vi "Autonomous Independent.vi"   [LabVIEW 2016]
doc: "This VI is called when autonomous begins, and will automatically be terminated when autonomous ends. You can carry out timed or sensor driven robot movement independently without needing to return to the caller."
uses:
  <vilib>/Rock Robotics/WPI/Utilities/WPI_GetSetVariantRefNum.vi
  <vilib>/Rock Robotics/Network Tables/NT Read String.vi
  <vilib>/Rock Robotics/Network Tables/NT Write Numeric Array.vi
panel:
  # "Be sure to right-click and choose Data Operations>>Make Current Value default if you want to save the array values with the VI"
types:
  T1 = typedef "WPI_JoystickDevRef.ctl" = cluster{"Device":T2}
  T2 = typedef "WPI_JoystickDeviceEnum.ctl" = enum16{"USB 0", "USB 1", "USB 2", "USB 3", "USB 4", "USB 5"}
  T3 = typedef "WPI_RobotDriveDevRef.ctl" = cluster{"DevStatus":errorcluster, "Motors[]":T4[], "Square Inputs":bool, "Max Output":dbl}
  T4 = typedef "WPI_MotorControlDeviceRef.ctl" = cluster{"DeviceStatus":errorcluster, "Type":T5, "PWM":cluster{"PWM Channel":T6, "DeadBand":T7}, "CAN":cluster{"Device Number":u8, "SetOutput VI Ref":variant, "GetOutput VI Ref":variant, "Enable VI Ref":variant, "Disable VI Ref":variant, "Data":variant}, "Invert":bool}
  T5 = typedef "WPI_MotorControlType.ctl" = enum16{"PWM", "CAN"}
  T6 = typedef "FPGA_DIOPWMChannel.ctl" = enum8{"PWM 0", "PWM 1", "PWM 2", "PWM 3", "PWM 4", "PWM 5", "PWM 6", "PWM 7", "PWM 8", "PWM 9", "PWM MXP 0", "PWM MXP 1", "PWM MXP 2", "PWM MXP 3", "PWM MXP 4", "PWM MXP 5", "PWM MXP 6", "PWM MXP 7", "PWM MXP 8", "PWM MXP 9", "Invalid"}
  T7 = typedef "WPI_PWMDeadband.ctl" = cluster{"Name":string, "maxPositivePwm":i32, "minPositivePwm":i32, "centerPwm":i32, "maxNegativePwm":i32, "minNegativePwm":i32, "angularRange":u16}
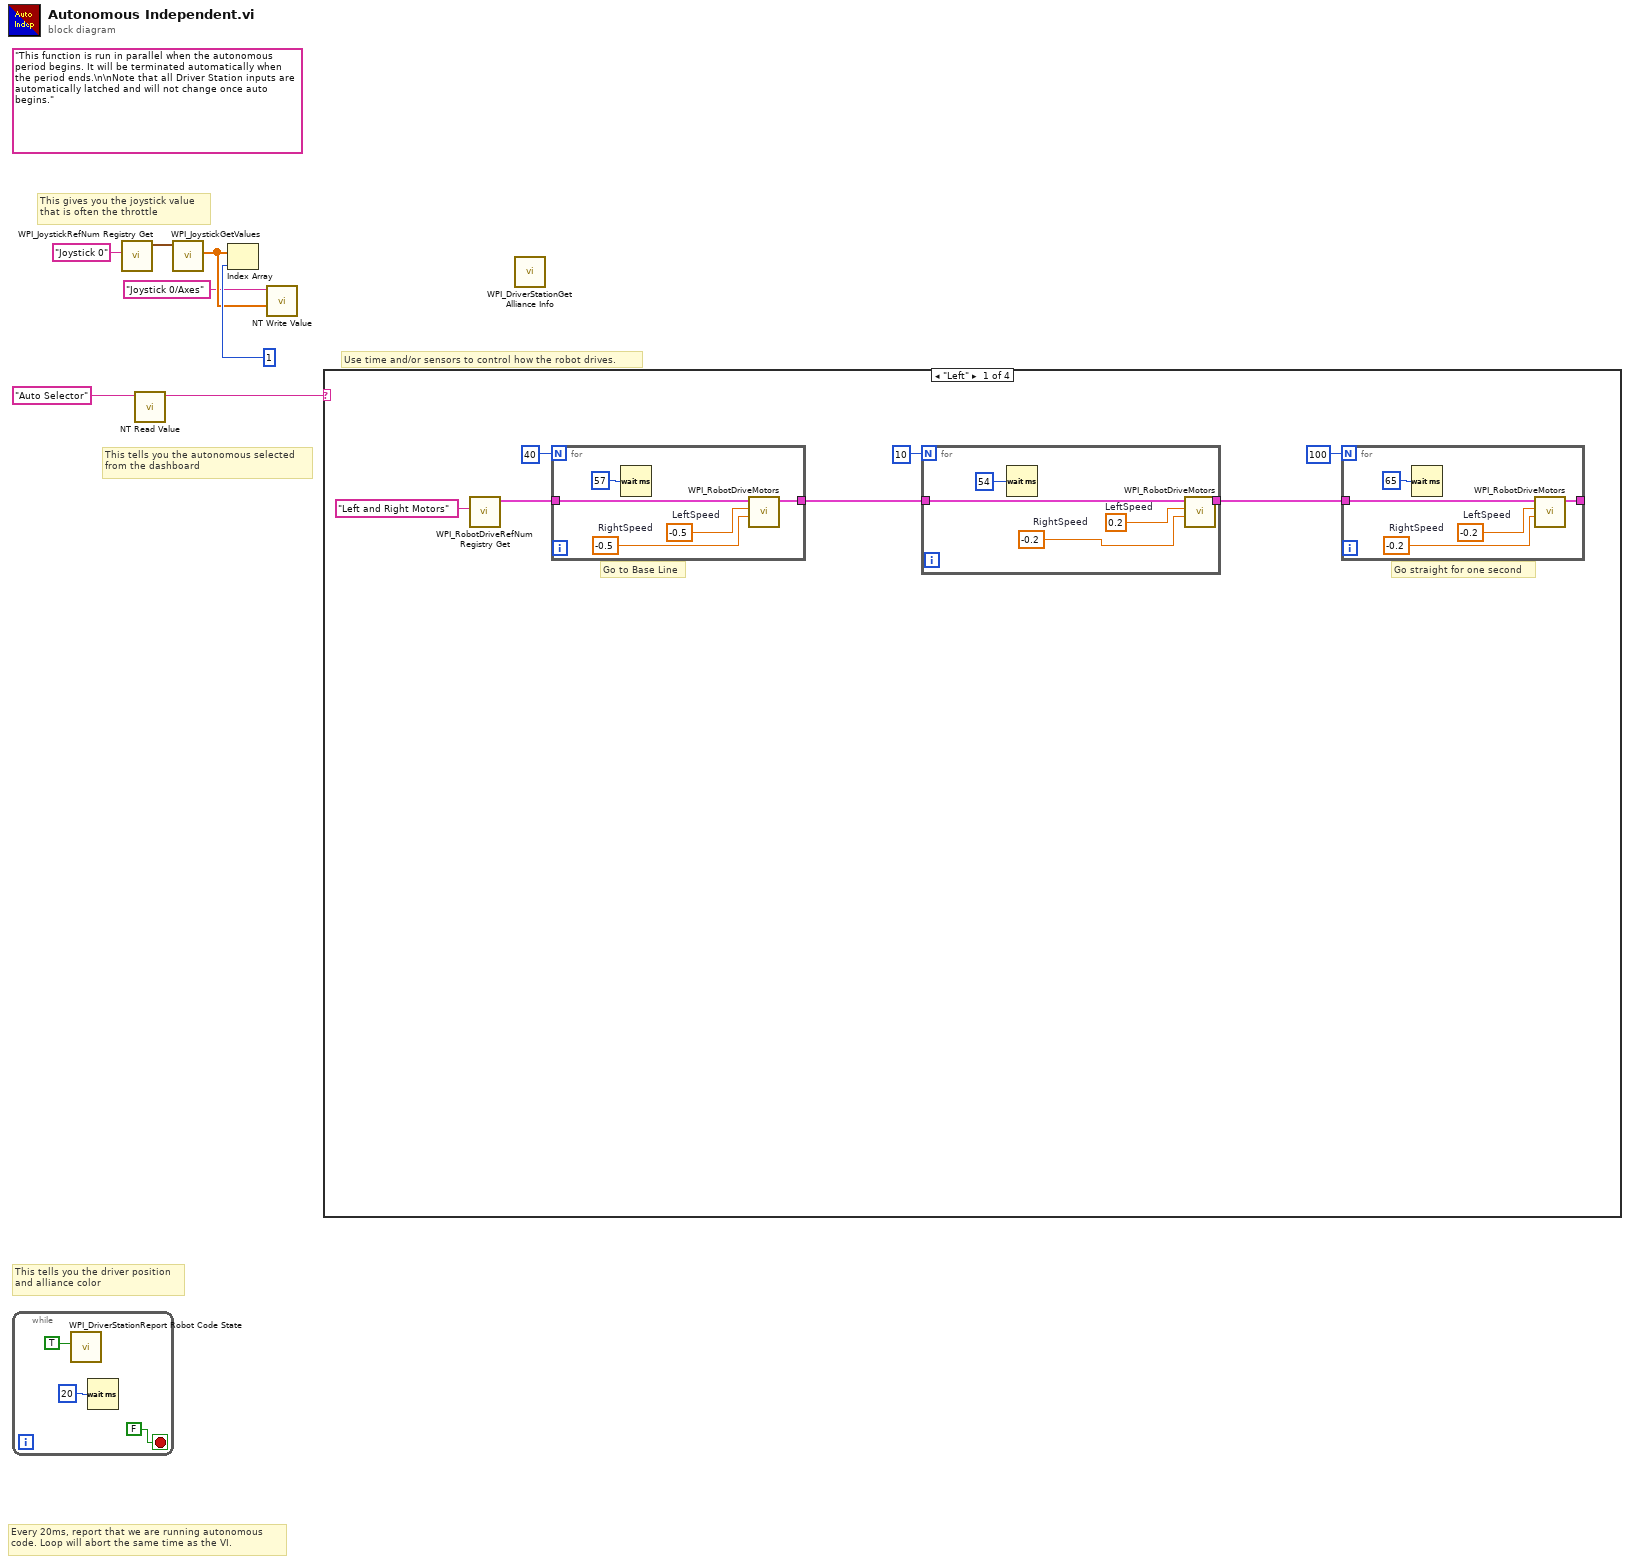
[diagram p0: block diagram]
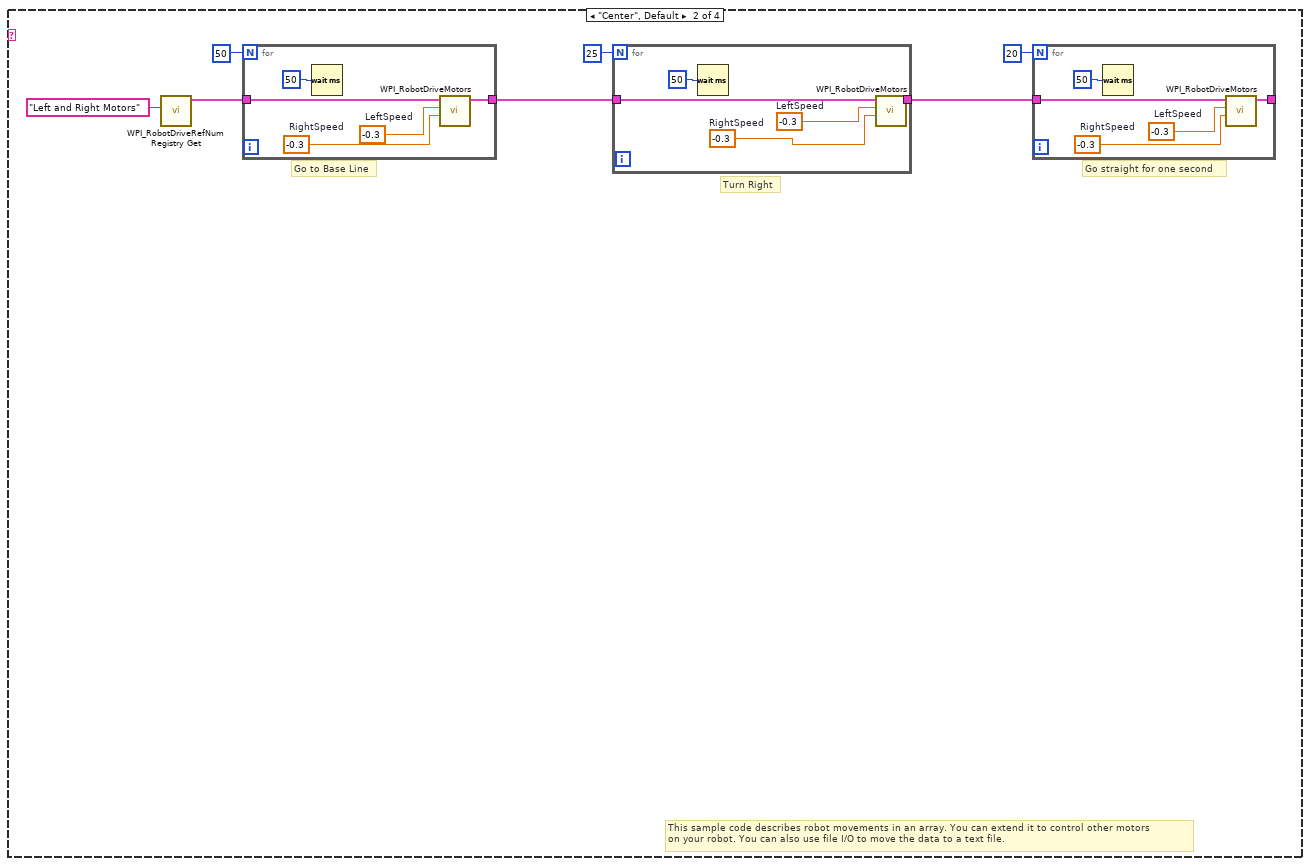
[diagram p2: hidden frame]
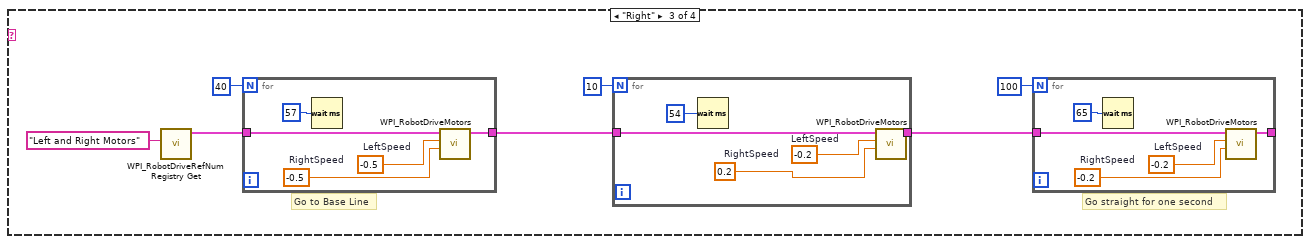
[diagram p3: hidden frame]
diagram:
  (unwired) "This function is run in parallel when the autonomous period begins. It will be terminated automatically when the period ends.\n\nNote that all Driver Station inputs are automatically latched and will not change once auto begins."
  # "This tells you the autonomous selected\nfrom the dashboard"
  # "Every 20ms, report that we are running autonomous\ncode. Loop will abort the same time as the VI."
  # "This gives you the joystick value\nthat is often the throttle"
  # "Use time and/or sensors to control how the robot drives."
  # "This tells you the driver position\nand alliance color"
  n1 = while {
    stop <- FALSE stop-if-true
    n2 = call <vilib>:"WPI_DriverStationReport Robot Code State.vi"("Autonomous"=TRUE) -> ()  [unwired: 10 in, 1 out]
    n3 = Wait (ms)(milliseconds to wait=u32 20) -> ()  [unwired: 1 out]
  }
  n4 = call <vilib>:"WPI_JoystickRefNum Registry Get.vi"("refnum name"="Joystick 0") -> ("JoystickDevRef"=w6:T1)  [unwired: 1 in, 9 out]
  n5 = call-poly <vilib>:"NT Read Value.vi"("Name"="Auto Selector") -> ("String"=w3:string)  [unwired: 9 in, 1 out]
  n6 = call <vilib>:"WPI_JoystickGetValues.vi"("JoystickDevRef"=w6) -> ("Axes"=w2:dbl[])  [unwired: 6 in, 4 out]
  n7 = Index Array(array=w2, index=1) -> ()  [unwired: 1 out]
  n8 = call-poly <vilib>:"NT Write Value.vi"("Numeric Array"=w2, "Name"="Joystick 0/Axes") -> ()  [unwired: 9 in, 1 out]
  n9 = case shown="\"Left\"" w3 {
    frame "Left" {
      # "Go straight for one second"
      # "Go to Base Line"
      n10 = call <vilib>:"WPI_RobotDriveRefNum Registry Get.vi"("refnum name"="Left and Right Motors") -> ("RobotDriveDevRef"=w16:T3)  [unwired: 1 in, 9 out]
      n11 = for {
        N: 40 -> [_]
        tunnel: w16 -> [w32]
        tunnel: [w28] -> w12
        w29 = -0.5  # RightSpeed
        w30 = -0.5  # LeftSpeed
        n12 = Wait (ms)(milliseconds to wait=u32 57) -> ()  [unwired: 1 out]
        n13 = call <vilib>:"WPI_RobotDriveMotors.vi"("RightSpeed"=w29, "LeftSpeed"=w30, "RobotDriveDevRef"=w32) -> ("RobotDriveDevRef"=w28:T3)  [unwired: 6 in, 2 out]
      }
      n14 = for {
        N: 10 -> [_]
        tunnel: w12 -> [w22]
        tunnel: [w18] -> w11
        w19 = -0.2  # RightSpeed
        w20 = 0.2  # LeftSpeed
        n15 = Wait (ms)(milliseconds to wait=u32 54) -> ()  [unwired: 1 out]
        n16 = call <vilib>:"WPI_RobotDriveMotors.vi"("RightSpeed"=w19, "LeftSpeed"=w20, "RobotDriveDevRef"=w22) -> ("RobotDriveDevRef"=w18:T3)  [unwired: 6 in, 2 out]
      }
      n17 = for {
        N: 100 -> [_]
        tunnel: w11 -> [w27]
        tunnel: [w23] -> _
        w24 = -0.2  # RightSpeed
        w25 = -0.2  # LeftSpeed
        n18 = Wait (ms)(milliseconds to wait=u32 65) -> ()  [unwired: 1 out]
        n19 = call <vilib>:"WPI_RobotDriveMotors.vi"("RightSpeed"=w24, "LeftSpeed"=w25, "RobotDriveDevRef"=w27) -> ("RobotDriveDevRef"=w23:T3)  [unwired: 6 in, 2 out]
      }
    }
    frame "Center", Default {
      # "Turn Right"
      # "Go straight for one second"
      # "Go to Base Line"
      # "This sample code describes robot movements in an array. You can extend it to control other motors\non your robot. You can also use file I/O to move the data to a text file."
      n20 = call <vilib>:"WPI_RobotDriveRefNum Registry Get.vi"("refnum name"="Left and Right Motors") -> ("RobotDriveDevRef"=w38:T3)  [unwired: 1 in, 9 out]
      n21 = for {
        N: 50 -> [_]
        tunnel: w38 -> [w54]
        tunnel: [w50] -> w34
        w51 = -0.3  # RightSpeed
        w52 = -0.3  # LeftSpeed
        n22 = Wait (ms)(milliseconds to wait=u32 50) -> ()  [unwired: 1 out]
        n23 = call <vilib>:"WPI_RobotDriveMotors.vi"("RightSpeed"=w51, "LeftSpeed"=w52, "RobotDriveDevRef"=w54) -> ("RobotDriveDevRef"=w50:T3)  [unwired: 6 in, 2 out]
      }
      n24 = for {
        N: 25 -> [_]
        tunnel: w34 -> [w44]
        tunnel: [w40] -> w33
        w41 = -0.3  # RightSpeed
        w42 = -0.3  # LeftSpeed
        n25 = Wait (ms)(milliseconds to wait=u32 50) -> ()  [unwired: 1 out]
        n26 = call <vilib>:"WPI_RobotDriveMotors.vi"("RightSpeed"=w41, "LeftSpeed"=w42, "RobotDriveDevRef"=w44) -> ("RobotDriveDevRef"=w40:T3)  [unwired: 6 in, 2 out]
      }
      n27 = for {
        N: 20 -> [_]
        tunnel: w33 -> [w49]
        tunnel: [w45] -> _
        w46 = -0.3  # RightSpeed
        w47 = -0.3  # LeftSpeed
        n28 = Wait (ms)(milliseconds to wait=u32 50) -> ()  [unwired: 1 out]
        n29 = call <vilib>:"WPI_RobotDriveMotors.vi"("RightSpeed"=w46, "LeftSpeed"=w47, "RobotDriveDevRef"=w49) -> ("RobotDriveDevRef"=w45:T3)  [unwired: 6 in, 2 out]
      }
    }
    frame "Right" {
      # "Go straight for one second"
      # "Go to Base Line"
      n30 = call <vilib>:"WPI_RobotDriveRefNum Registry Get.vi"("refnum name"="Left and Right Motors") -> ("RobotDriveDevRef"=w56:T3)  [unwired: 1 in, 9 out]
      n31 = for {
        N: 40 -> [_]
        tunnel: w56 -> [w76]
        tunnel: [w72] -> w60
        w73 = -0.5  # RightSpeed
        w74 = -0.5  # LeftSpeed
        n32 = Wait (ms)(milliseconds to wait=u32 57) -> ()  [unwired: 1 out]
        n33 = call <vilib>:"WPI_RobotDriveMotors.vi"("RightSpeed"=w73, "LeftSpeed"=w74, "RobotDriveDevRef"=w76) -> ("RobotDriveDevRef"=w72:T3)  [unwired: 6 in, 2 out]
      }
      n34 = for {
        N: 10 -> [_]
        tunnel: w60 -> [w66]
        tunnel: [w62] -> w61
        w63 = 0.2  # RightSpeed
        w64 = -0.2  # LeftSpeed
        n35 = Wait (ms)(milliseconds to wait=u32 54) -> ()  [unwired: 1 out]
        n36 = call <vilib>:"WPI_RobotDriveMotors.vi"("RightSpeed"=w63, "LeftSpeed"=w64, "RobotDriveDevRef"=w66) -> ("RobotDriveDevRef"=w62:T3)  [unwired: 6 in, 2 out]
      }
      n37 = for {
        N: 100 -> [_]
        tunnel: w61 -> [w71]
        tunnel: [w67] -> _
        w68 = -0.2  # RightSpeed
        w69 = -0.2  # LeftSpeed
        n38 = Wait (ms)(milliseconds to wait=u32 65) -> ()  [unwired: 1 out]
        n39 = call <vilib>:"WPI_RobotDriveMotors.vi"("RightSpeed"=w68, "LeftSpeed"=w69, "RobotDriveDevRef"=w71) -> ("RobotDriveDevRef"=w67:T3)  [unwired: 6 in, 2 out]
      }
    }
    frame "Your Turn" {
    }
  }
  n40 = call <vilib>:"WPI_DriverStationGet Alliance Info.vi"() -> ()  [unwired: 12 out]
